vi "Acquire - Flush AT Serial Buffer.vi"(8 "Error In":errorcluster, 11 "Settings In":T1) -> (0 "Error Out":errorcluster, 3 "Settings Out":T1)   [LabVIEW 2019, in "cRIO Acquisition.lvlib"]
uses:
  cRIO Acquisition.lvlib
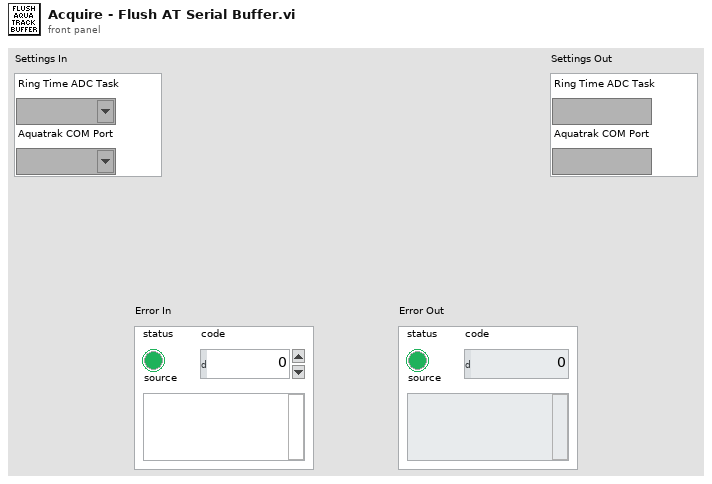
[diagram p1: front panel]
types:
  T1 = cluster{"Ring Time ADC Task":refnum<k21>, "Aquatrak COM Port":refnum<visa-resource-name>}
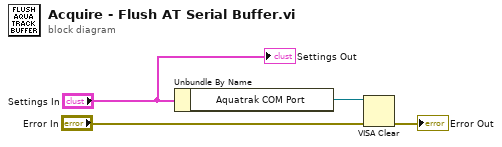
[diagram p0: block diagram]
diagram:
  n1 = Unbundle By Name("Settings In") -> ("Aquatrak COM Port"=w4:refnum<visa-resource-name>)
  n2 = VISA Clear(VISA resource name=w4, error in (no error)="Error In") -> (error out=→"Error Out":errorcluster)  [unwired: 1 out]
  "Settings Out" <- "Settings In"
